vi "Force Reload_Write.vi"(8 "error in (no error)":errorcluster, 10 "Force Reload?(F)":bool, 11 "Dependency Source_VIPM in":refnum<class "Dependency Source_VIPM.lvclass">) -> (0 "error out":errorcluster, 3 "Dependency Source_VIPM out":refnum<class "Dependency Source_VIPM.lvclass">)   [LabVIEW 2019, in "Project.Dependencies Finder.lvlib" / "Dependency Source_VIPM.lvclass"]
uses:
  Dependency Source_VIPM.lvclass
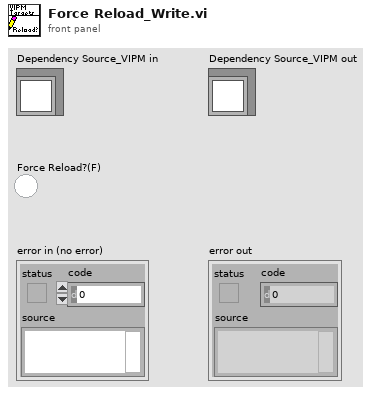
[diagram p1: front panel]
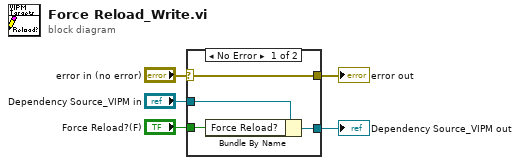
[diagram p0: block diagram]
diagram:
  n1 = case shown="No Error" "error in (no error)" {
    selector: "error in (no error)" -> [w9 w10]
    tunnel: [w9 w10] -> w4
    tunnel: [w7 w11] -> w2
    tunnel: "Dependency Source_VIPM in" -> [w8 w11]
    tunnel: "Force Reload?(F)" -> [w6 _]
    frame No Error {
      n2 = Bundle By Name(cluster=w8, "Force Reload?"=w6) -> (w7:refnum<class "Dependency Source_VIPM.lvclass">)
    }
    frame Error {
    }
  }
  "error out" <- w4
  "Dependency Source_VIPM out" <- w2
